vi "Read Configuration Parameters.vi"(8 "error in (no error)":errorcluster, 10 "refnum":T1, 11 "Example Configuration Dialog in":refnum<class "Inclinometer Configuration.lvclass">) -> (0 "error out":errorcluster, 2 "refnum out":T1, 3 "Example Configuration Dialog out":refnum<class "Inclinometer Configuration.lvclass">)   [LabVIEW 2016, in "Hardware.lvlib" / "Inclinometer.lvlib" / "Inclinometer Configuration.lvclass"]
uses:
  <userlib>/Common Components/Hardware/Inclinometer/Inclinometer Config/Inclinometer Configuration.lvclass
  <vilib>/Utility/config.llb/Config Data RefNum.ctl
  <userlib>/Common Components/Hardware/Inclinometer/Inclinometer Config/Inclinometer Configuration.lvclass/Inclinometer Configuration.ctl
  <userlib>/Common Components/Hardware/Abstract Hardware/Hardware.lvclass/Hardware.ctl
  <userlib>/Common Components/Hardware/DevInfo/DevInfo.lvclass/DevInfo.ctl
  <userlib>/Common Components/Hardware/DevInfo/Read HW Type.vi
  <userlib>/Common Components/Hardware/DevInfo/Read Device Name.vi
  <userlib>/Common Components/Hardware/DevInfo/Read COMM Address.vi
  <userlib>/Common Components/Hardware/DevInfo/Read Sub-COMM Address.vi
  <userlib>/Common Components/Hardware/DevInfo/Write HW Type.vi
  <userlib>/Common Components/Hardware/DevInfo/Write Device Name.vi
  <userlib>/Common Components/Hardware/DevInfo/Write COMM Address.vi
  <userlib>/Common Components/Hardware/DevInfo/Write Sub-COMM Address.vi
  <userlib>/Common Components/Hardware/Abstract Hardware/Write DevInfo.vi
  <userlib>/Common Components/Hardware/Inclinometer/Inclinometer Config/Accessors/Write Inclinometer Obj.vi
  <userlib>/Common Components/Hardware/Inclinometer/Inclinometer Config/Accessors/Read Inclinometer Obj.vi
  <userlib>/Common Components/Hardware/Abstract Hardware/Read Label.vi
  <userlib>/Common Components/Hardware/Abstract Hardware/Read DevInfo.vi
  <userlib>/Common Components/Hardware/Inclinometer/Inclinometer/Inclinometer.lvclass
  C:/Program Files (x86)/National Instruments/LabVIEW 2016/user.lib/Common Components/Hardware/Abstract Hardware/Hardware.lvclass
  <userlib>/Common Components/Hardware/DevInfo/DevInfo.lvclass
  <userlib>/Configuration Dialog Actor/Configuration.lvclass
  <vilib>/Utility/config.llb/NI_LVConfig.lvlib
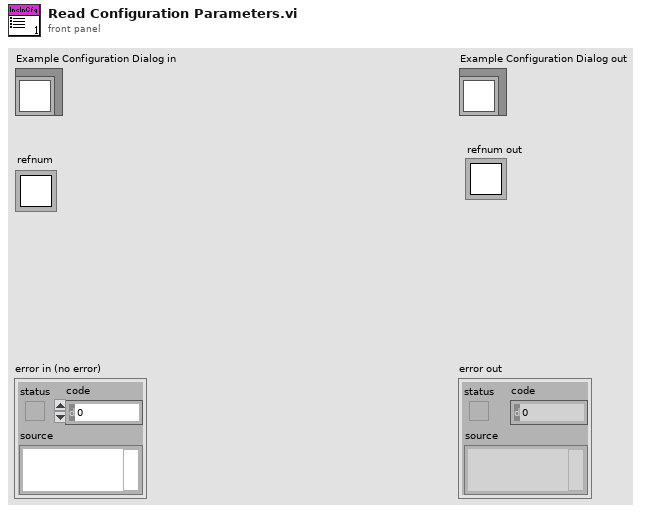
[diagram p1: front panel]
types:
  T1 = typedef "NI_LVConfig.lvlib/Config Data RefNum.ctl" = refnum<k1>
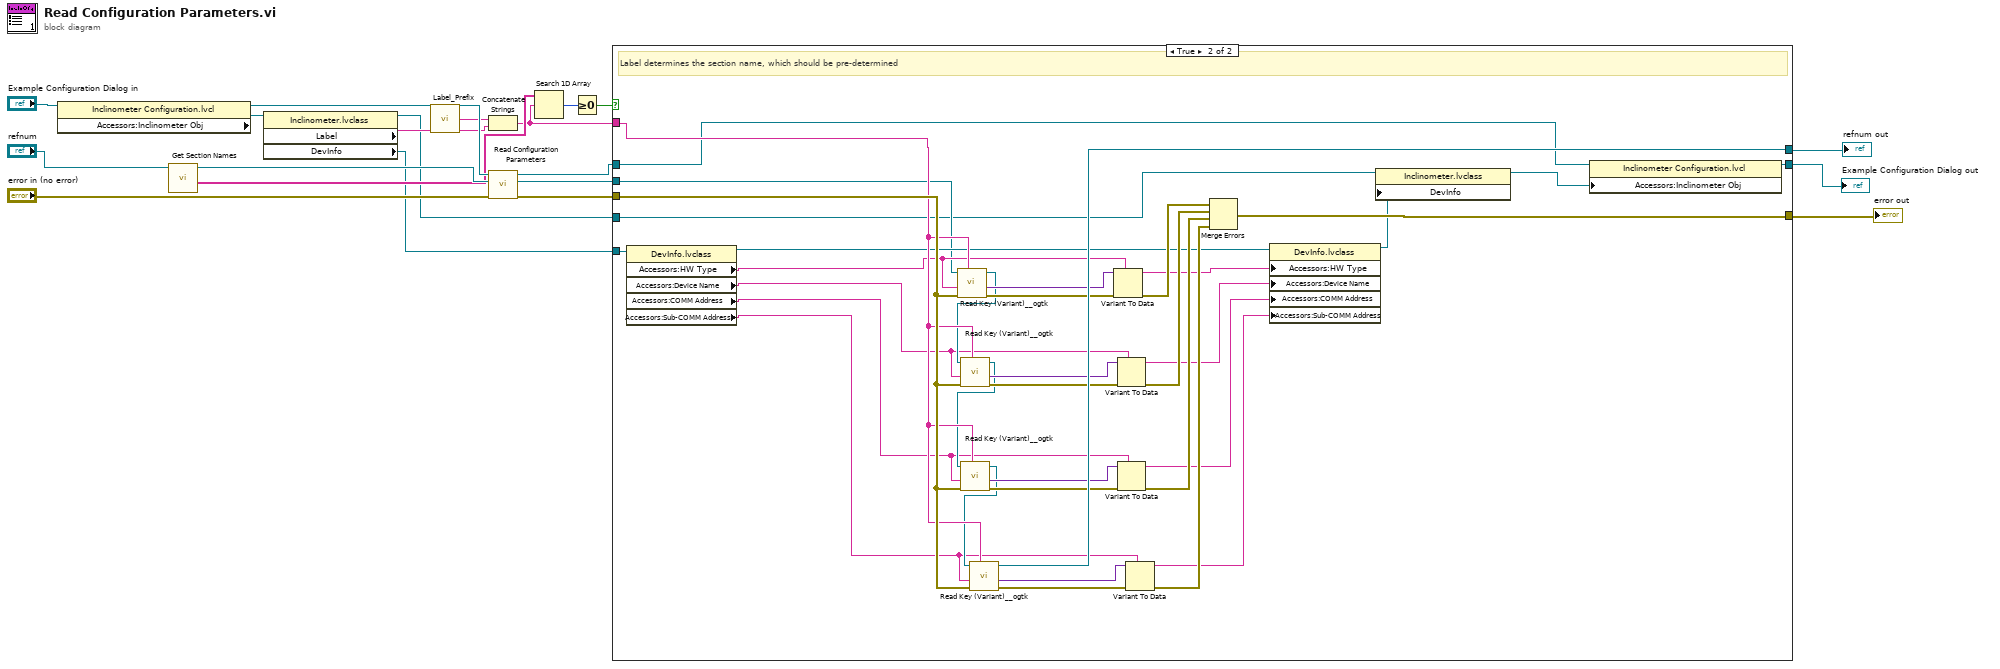
[diagram p0: block diagram]
diagram:
  n1 = property class="Inclinometer Configuration.lvcl"(reference="Example Configuration Dialog in") -> (reference out=w11:refnum<class "Inclinometer Configuration.lvclass">, "Accessors:Inclinometer Obj"=w9:refnum<class "Inclinometer.lvclass">)  [unwired: 1 in, 1 out]
  n2 = call <vilib>:"Get Section Names.vi"("refnum"="refnum") -> ("section names"=w7:string[], "refnum out"=w8:T1)  [unwired: 8 in, 1 out]
  n3 = property class="Inclinometer.lvclass"(reference=w9) -> (reference out=w2:refnum<class "Inclinometer.lvclass">, "Label"=w3:string, "DevInfo"=w1:refnum<class "DevInfo.lvclass">)  [unwired: 1 in, 1 out]
  n4 = call <userlib>:"Label_Prefix.vi"() -> ("Label Prefix String"=w10:string)
  n5 = Concatenate Strings(w10, w3) -> (w6:string)
  n6 = call-parent "Read Configuration Parameters.vi"("error in (no error)"="error in (no error)", "refnum"=w8, "Configuration in"=w11) -> ("error out"=w17:errorcluster, "refnum out"=w18:T1, "Configuration out"=w16:refnum<class "Inclinometer Configuration.lvclass">)  [unwired: 6 in]
  n7 = Search 1D Array(1D array=w7, element=w6) -> (index of element=w5:i32)  [unwired: 1 in]
  n8 = Greater Or Equal To 0?(x=w5) -> (x >= 0?=w4:bool)
  n9 = case shown="True" w4 {
    tunnel: w18 -> [w22 w25]
    tunnel: w17 -> [w21 w58]
    tunnel: w16 -> [w23 w27]
    tunnel: [w23 w28] -> w15
    tunnel: [w22 w56] -> w14
    tunnel: [w21 w55] -> w13
    tunnel: w6 -> [_ w57]
    tunnel: w2 -> [_ w24]
    tunnel: w1 -> [_ w39]
    frame False {
    }
    frame True {
      # "Label determines the section name, which should be pre-determined"
      n10 = property class="DevInfo.lvclass"(reference=w39) -> (reference out=w34:refnum<class "DevInfo.lvclass">, "Accessors:HW Type"=w38:string, "Accessors:Device Name"=w37:string, "Accessors:COMM Address"=w36:string, "Accessors:Sub-COMM Address"=w35:string)  [unwired: 1 in, 1 out]
      n11 = call <userlib>:"Read Key (Variant)__ogtk.vi"("section"=w57, "error in (no error)"=w58, "type"=w38, "refnum"=w25) -> ("error out"=w53:errorcluster, "key-value"=w54:variant, "refnum out"=w46:T1)  [unwired: 4 in, 1 out]
      n12 = call <userlib>:"Read Key (Variant)__ogtk.vi"("section"=w57, "error in (no error)"=w58, "type"=w37, "refnum"=w46) -> ("error out"=w51:errorcluster, "key-value"=w52:variant, "refnum out"=w45:T1)  [unwired: 4 in, 1 out]
      n13 = call <userlib>:"Read Key (Variant)__ogtk.vi"("section"=w57, "error in (no error)"=w58, "type"=w36, "refnum"=w45) -> ("error out"=w49:errorcluster, "key-value"=w50:variant, "refnum out"=w44:T1)  [unwired: 4 in, 1 out]
      n14 = call <userlib>:"Read Key (Variant)__ogtk.vi"("section"=w57, "error in (no error)"=w58, "type"=w35, "refnum"=w44) -> ("error out"=w47:errorcluster, "key-value"=w48:variant, "refnum out"=w56:T1)  [unwired: 4 in, 1 out]
      n15 = Variant To Data(error in=w53, type=w38, Variant=w54) -> (data=w33:string, error out=w43:errorcluster)
      n16 = Variant To Data(error in=w51, type=w37, Variant=w52) -> (data=w32:string, error out=w42:errorcluster)
      n17 = Variant To Data(error in=w49, type=w36, Variant=w50) -> (data=w31:string, error out=w41:errorcluster)
      n18 = Variant To Data(error in=w47, type=w35, Variant=w48) -> (data=w30:string, error out=w40:errorcluster)
      n19 = Merge Errors(w43, w42, w41, w40) -> (w55:errorcluster)
      n20 = property class="DevInfo.lvclass"(reference=w34, "Accessors:HW Type"=w33, "Accessors:Device Name"=w32, "Accessors:COMM Address"=w31, "Accessors:Sub-COMM Address"=w30) -> (reference out=w29:refnum<class "DevInfo.lvclass">)  [unwired: 1 in, 1 out]
      n21 = property class="Inclinometer.lvclass"(reference=w24, "DevInfo"=w29) -> (reference out=w26:refnum<class "Inclinometer.lvclass">)  [unwired: 1 in, 1 out]
      n22 = property class="Inclinometer Configuration.lvcl"(reference=w27, "Accessors:Inclinometer Obj"=w26) -> (reference out=w28:refnum<class "Inclinometer Configuration.lvclass">)  [unwired: 1 in, 1 out]
    }
  }
  "Example Configuration Dialog out" <- w15
  "error out" <- w13
  "refnum out" <- w14
